vi "Apply tau delay.vi"(0 "reference in":refnum<class "Fcurve.lvclass">, 5 "error in (no error)":errorcluster, 8 "Section":T1) -> (14 "reference out":refnum<class "Fcurve.lvclass">, 15 "Dec factor":i32, 16 "# of samples":i32, 19 "error out":errorcluster)   [LabVIEW 2019, in "Fcurve.lvclass"]
doc: "This takes to account the delay time of the slowest time constant of the afm control system"
uses:
  Fcurve.lvclass
  Fcurve sections.ctl
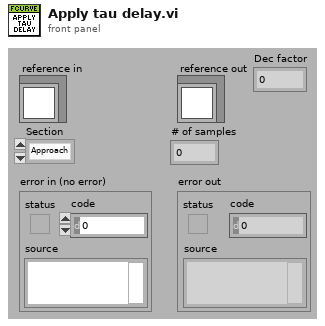
[diagram p1: front panel]
types:
  T1 = typedef "Fcurve.lvclass/Fcurve sections.ctl" = enum16{"Approach", "Contact", "Retract"}
  T2 = typedef "Fcurve.lvclass/ObjectAttributes.ctl" = cluster{"MyAttribute":dbl, "Fcurve Metadata":T3, "Contact Spread of dev":dbl, "Tau Delay (ms)":dbl, "Points of contact":dbl, "Def_wfm":cluster{"Max":dbl, "Min":dbl}, "Zpos_wfm":cluster{"Max":dbl, "Min":dbl}, "Contact stat?":bool, "Real AI dt (s)":dbl, "Decimation":cluster{"App":cluster{"Dec":i32, "apply":bool}, "Con":cluster{"Dec":i32, "apply":bool}, "Ret":cluster{"Dec":i32, "apply":bool}}, "Segment def[0]":dbl, "Segment Zpos[0]":dbl, "Raw Datum":waveform(dbl)[], "Group metadata":T4, "M_data obj":refnum<class "metadata.lvclass">, "Channel name(s)":string[], "Segment fcurve data":cluster{"X":dbl[], "Y":dbl[]}[], "Segment duration":cluster{"Start":i32, "Duration":i32}[], "Segment info":T5[], "Segment durations (S)":dbl[], "Segments Maxmin":T7[]}
  T3 = typedef "Fcurve.lvclass/Metadata.ctl" = cluster{"dt (us)":dbl, "Dec Factor":dbl, "Z piezo Sensitivity (nm/V)":dbl, "K (N/m)":dbl, "Sp (V)":dbl, "Contact (ms)":dbl, "Zpos contact":dbl, "Vel_app (nm/s)":dbl, "Vel_ret (nm/s)":dbl, "deltaV (nm)":dbl, "Def_V0 (v)":dbl, "Piezo gain":dbl, "invOLS (nm/V)":dbl}
  T4 = typedef "TDMS_DataHandler.lvclass/Fcurve Meta data.ctl" = cluster{"property names":string[], "property values":variant[]}
  T5 = typedef "Fcurve.lvclass/Fcurve segments --cluster.ctl" = cluster{"type":T6, "nb points":i32, "dec factor":u32, "sampling rate (S/s)":u32}
  T6 = typedef "metadata.lvclass/Segment type--combobox.ctl" = string
  T7 = typedef "Fcurve.lvclass/Segment MaxMin --cluster.ctl" = cluster{"Def":cluster{"max value":dbl, "min value":dbl}, "Zpos":cluster{"max value":dbl, "min value":dbl}}
  T8 = cluster{"App":cluster{"Dec":i32, "apply":bool}, "Con":cluster{"Dec":i32, "apply":bool}, "Ret":cluster{"Dec":i32, "apply":bool}}
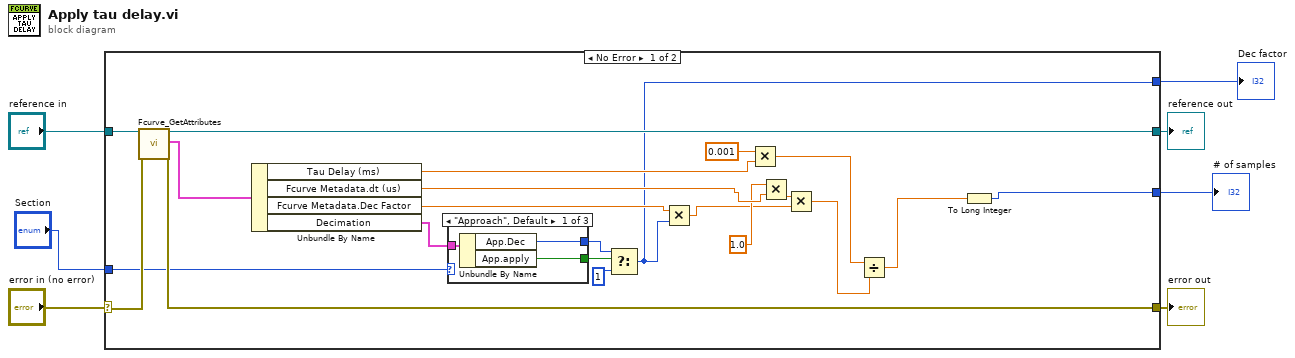
[diagram p0: block diagram]
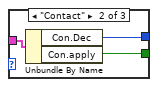
[diagram p2: hidden frame]
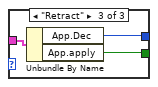
[diagram p3: hidden frame]
diagram:
  n1 = case shown="No Error" "error in (no error)" {
    selector: "error in (no error)" -> [w27 w40]
    tunnel: [w26 w40] -> w6
    tunnel: [w28 w39] -> w4
    tunnel: "reference in" -> [w29 w39]
    tunnel: "Section" -> [w14 _]
    tunnel: [w9 _] -> w2
    tunnel: [w8 _] -> w1
    frame No Error {
      n2 = call "Fcurve_GetAttributes.vi"("reference in"=w29, "error in (no error)"=w27) -> ("reference out"=w28:refnum<class "Fcurve.lvclass">, "attributes"=w25:T2, "error out"=w26:errorcluster)  [unwired: 14 in, 1 out]
      n3 = Unbundle By Name(w25) -> ("Tau Delay (ms)"=w23:dbl, "Fcurve Metadata.dt (us)"=w20:dbl, "Fcurve Metadata.Dec Factor"=w17:dbl, "Decimation"=w13:T8)
      n4 = case shown="\"Approach\", Default" w14 {
        tunnel: w13 -> [w32 w35 w38]
        tunnel: [w31 w33 w36] -> w11
        tunnel: [w30 w34 w37] -> w10
        frame "Approach", Default {
          n5 = Unbundle By Name(w32) -> ("App.Dec"=w30:i32, "App.apply"=w31:bool)
        }
        frame "Contact" {
          n6 = Unbundle By Name(w35) -> ("Con.Dec"=w34:i32, "Con.apply"=w33:bool)
        }
        frame "Retract" {
          n7 = Unbundle By Name(w38) -> ("App.Dec"=w37:i32, "App.apply"=w36:bool)
        }
      }
      n8 = Select(t=w10, s=w11, f=1) -> (s? t:f=w9:i32)
      n9 = Multiply(x=w17, y=w9) -> (x*y=w16:dbl)
      n10 = Multiply(x=0.001, y=w23) -> (x*y=w21:dbl)
      n11 = Multiply(x=1.0, y=w20) -> (x*y=w18:dbl)
      n12 = Multiply(x=w18, y=w16) -> (x*y=w24:dbl)
      n13 = Divide(x=w21, y=w24) -> (x/y=w15:dbl)
      n14 = To Long Integer(number=w15) -> (32bit integer=w8:i32)
    }
    frame Error {
    }
  }
  "error out" <- w6
  "reference out" <- w4
  "Dec factor" <- w2
  "# of samples" <- w1
